vi "strain_fgv.vi"(7 "cmd":T1, 8 "error in":errorcluster) -> (0 "error out":errorcluster, 3 "data":waveform(dbl)[](array[waveform]) caption="데이터")   [LabVIEW 2013]
uses:
  ctl/strain_ctl.ctl
  <vilib>/DAQmx/read.llb/DAQmx Read (Analog 1D Wfm NChan NSamp).vi
  <vilib>/DAQmx/miscellaneous.llb/DAQmx Fill In Error Info.vi
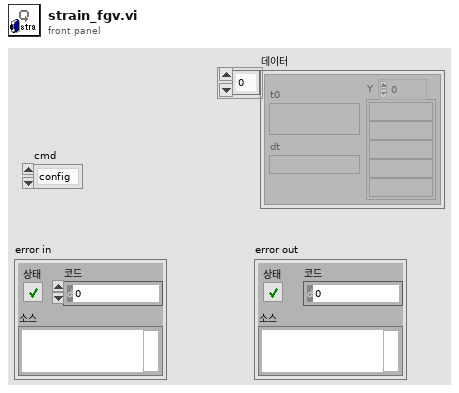
[diagram p1: front panel]
types:
  T1 = typedef "strain_ctl.ctl" = enum16{"config", "start", "read", "close"}
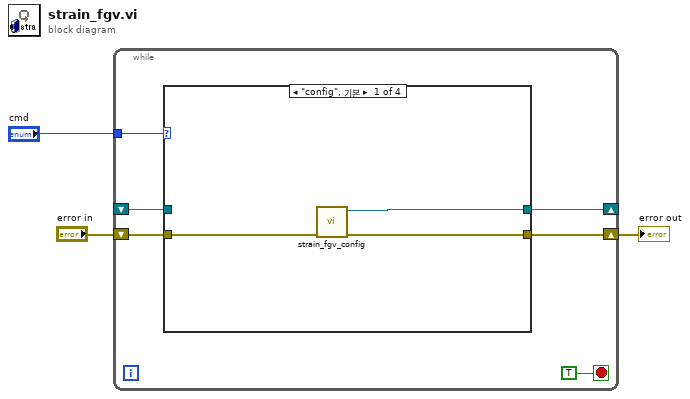
[diagram p0: block diagram]
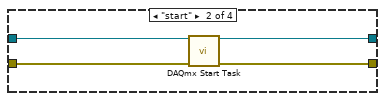
[diagram p2: hidden frame]
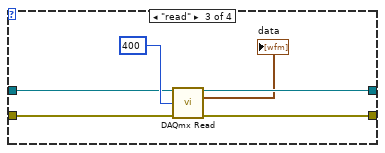
[diagram p3: hidden frame]
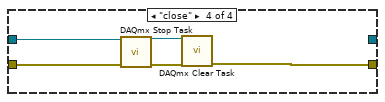
[diagram p4: hidden frame]
diagram:
  n1 = while {
    tunnel: "cmd" -> [w8]
    shift-right: [w6] -> _
    shift-left: _ -> [w5]
    shift-right: [w7] -> w2
    shift-left: "error in" -> [w4]
    stop <- TRUE stop-if-true
    n2 = case shown="\"config\", 기본" w8 {
      tunnel: [w11 w14 w20 w23] -> w7
      tunnel: [w12 w13 w21 _] -> w6
      tunnel: w5 -> [_ w15 w19 w24]
      tunnel: w4 -> [w10 w16 w18 w25]
      frame "config", Default {
        n3 = call "strain_fgv_config.vi"("error in"=w10) -> ("error out"=w11:errorcluster, "task out"=w12:refnum<k21>)  [unwired: 9 in]
      }
      frame "start" {
        n4 = call <vilib>:"DAQmx Start Task.vi"("task/channels in"=w15, "error in"=w16) -> ("task out"=w13:refnum<k21>, "error out"=w14:errorcluster)  [unwired: 12 in]
      }
      frame "read" {
        n5 = call-poly <vilib>:"DAQmx Read.vi"("task/channels in"=w19, "number of samples per channel"=400, "error in"=w18) -> ("task out"=w21:refnum<k21>, "data"=→"data":waveform(dbl)[], "error out"=w20:errorcluster)  [unwired: 10 in]
      }
      frame "close" {
        n6 = call <vilib>:"DAQmx Stop Task.vi"("task/channels in"=w24, "error in"=w25) -> ("task out"=w26:refnum<k21>, "error out"=w27:errorcluster)  [unwired: 12 in]
        n7 = call <vilib>:"DAQmx Clear Task.vi"("task in"=w26, "error in"=w27) -> ("error out"=w23:errorcluster)  [unwired: 13 in]
      }
    }
  }
  "error out" <- w2
